vi "Convert Test Profile.vi"(0 "Test Profile":T5[](array[typedef]) {"Pump Cmds"."Pump 6\nCmd" min=0 format="%#.1f"; "Pump Cmds"."Pump 5\nCmd" min=0 format="%#.1f"; "Pump Cmds"."Pump 4\nCmd" min=0 format="%#.1f"; "Pump Cmds"."Pump 3\nCmd" min=0 format="%#.1f"; "Pump Cmds"."Pump 2\nCmd" min=0 format="%#.1f"; "Pump Cmds"."Pump 1\nCmd" min=0 format="%#.1f"; "Temp\nCmd" min=-60 max=100; "Pressure\nCmd" max=20; "PS\nCmd" min=0 max=20 format="%#.2f"; "Time (s)" min=0.0 step=0.01 format="%#.2g"}, 5 "App Config":T7={"Location"="", "Profiles Path"=path "", "Current Profile"="", "CA Number"="", "Controller Type:"=enum."Kuhnke", "Stagger Time (ms)"=0, "Tank 1 Fuel"="", "Tank 2 Fuel"="", "Serial Numbers"={"Position 1 SN"="", "Position 2 SN"="", "Poaition 3 SN"="", "Position 4 SN"="", "Position 5 SN"="", "Position 6 SN"=""}, "Pumps Present"={"Pump 1"=FALSE, "Pump 2"=FALSE, "Pump 3"=FALSE, "Pump 4"=FALSE, "Pump 5"=FALSE, "Pump 6"=FALSE}, "VoltCtrlRef"="", "VoltageSelect"=FALSE, "Watlow Present"=FALSE, "Temp 1"=0, "Temp 2"=0, "Voltage Scale"={"V_FFm"=10.0, "V_FFb"=0.0}, "Pressure Scale"={"Pres_FFm"=0.0, "Pres_FFb"=0.0}, "Temp Format"=0, "Temp Tolerance"=0.0, "Target Voltage"=0.0, "Target Pressure"=0.0, "Data Log Init"={"Data Path"=path "", "Data Log Rate (S/s)"=0, "AKLH Rate (Hours/S)"=0.0, "Sync Time Offset (min)"=0, "IP Last 3"=0, "WebDAV IP"=""}, "Email Handler IP"="", "ADC Check"=FALSE, "3 Pump Tank"=FALSE, "Freq Flow?"=FALSE, "Profile Temp Control"=FALSE, "Read Controller Diag"=FALSE, "FFT Min Freq."=0, "FFT Max Freq."=0, "Speed by Current"=FALSE, "Watlow is F4T?"=FALSE, "Test Stop Time"=0.0, "Stop Time Enable"=TRUE, "Timers Include Off-Time"=FALSE, "Pump Timer Email"={"Enable"=FALSE, "Hour to Send"=0}}, 7 "Controller Config":T1) -> (4 "Test Profile (FPGA)":T4[](array[typedef]))   [LabVIEW 2019]
uses:
  Type Defs/App Config.ctl
  Type Defs/Controller Names.ctl
  Data Logger/Data Log Init.ctl
  Type Defs/Pump Timer Email.ctl
  Type Defs/Test Step.ctl
  Type Defs/Pump Cmds.ctl
  Type Defs/Test Step (FPGA).ctl
  Controls/Controller Config.ctl
  Type Defs/Diagnostic Mode.ctl
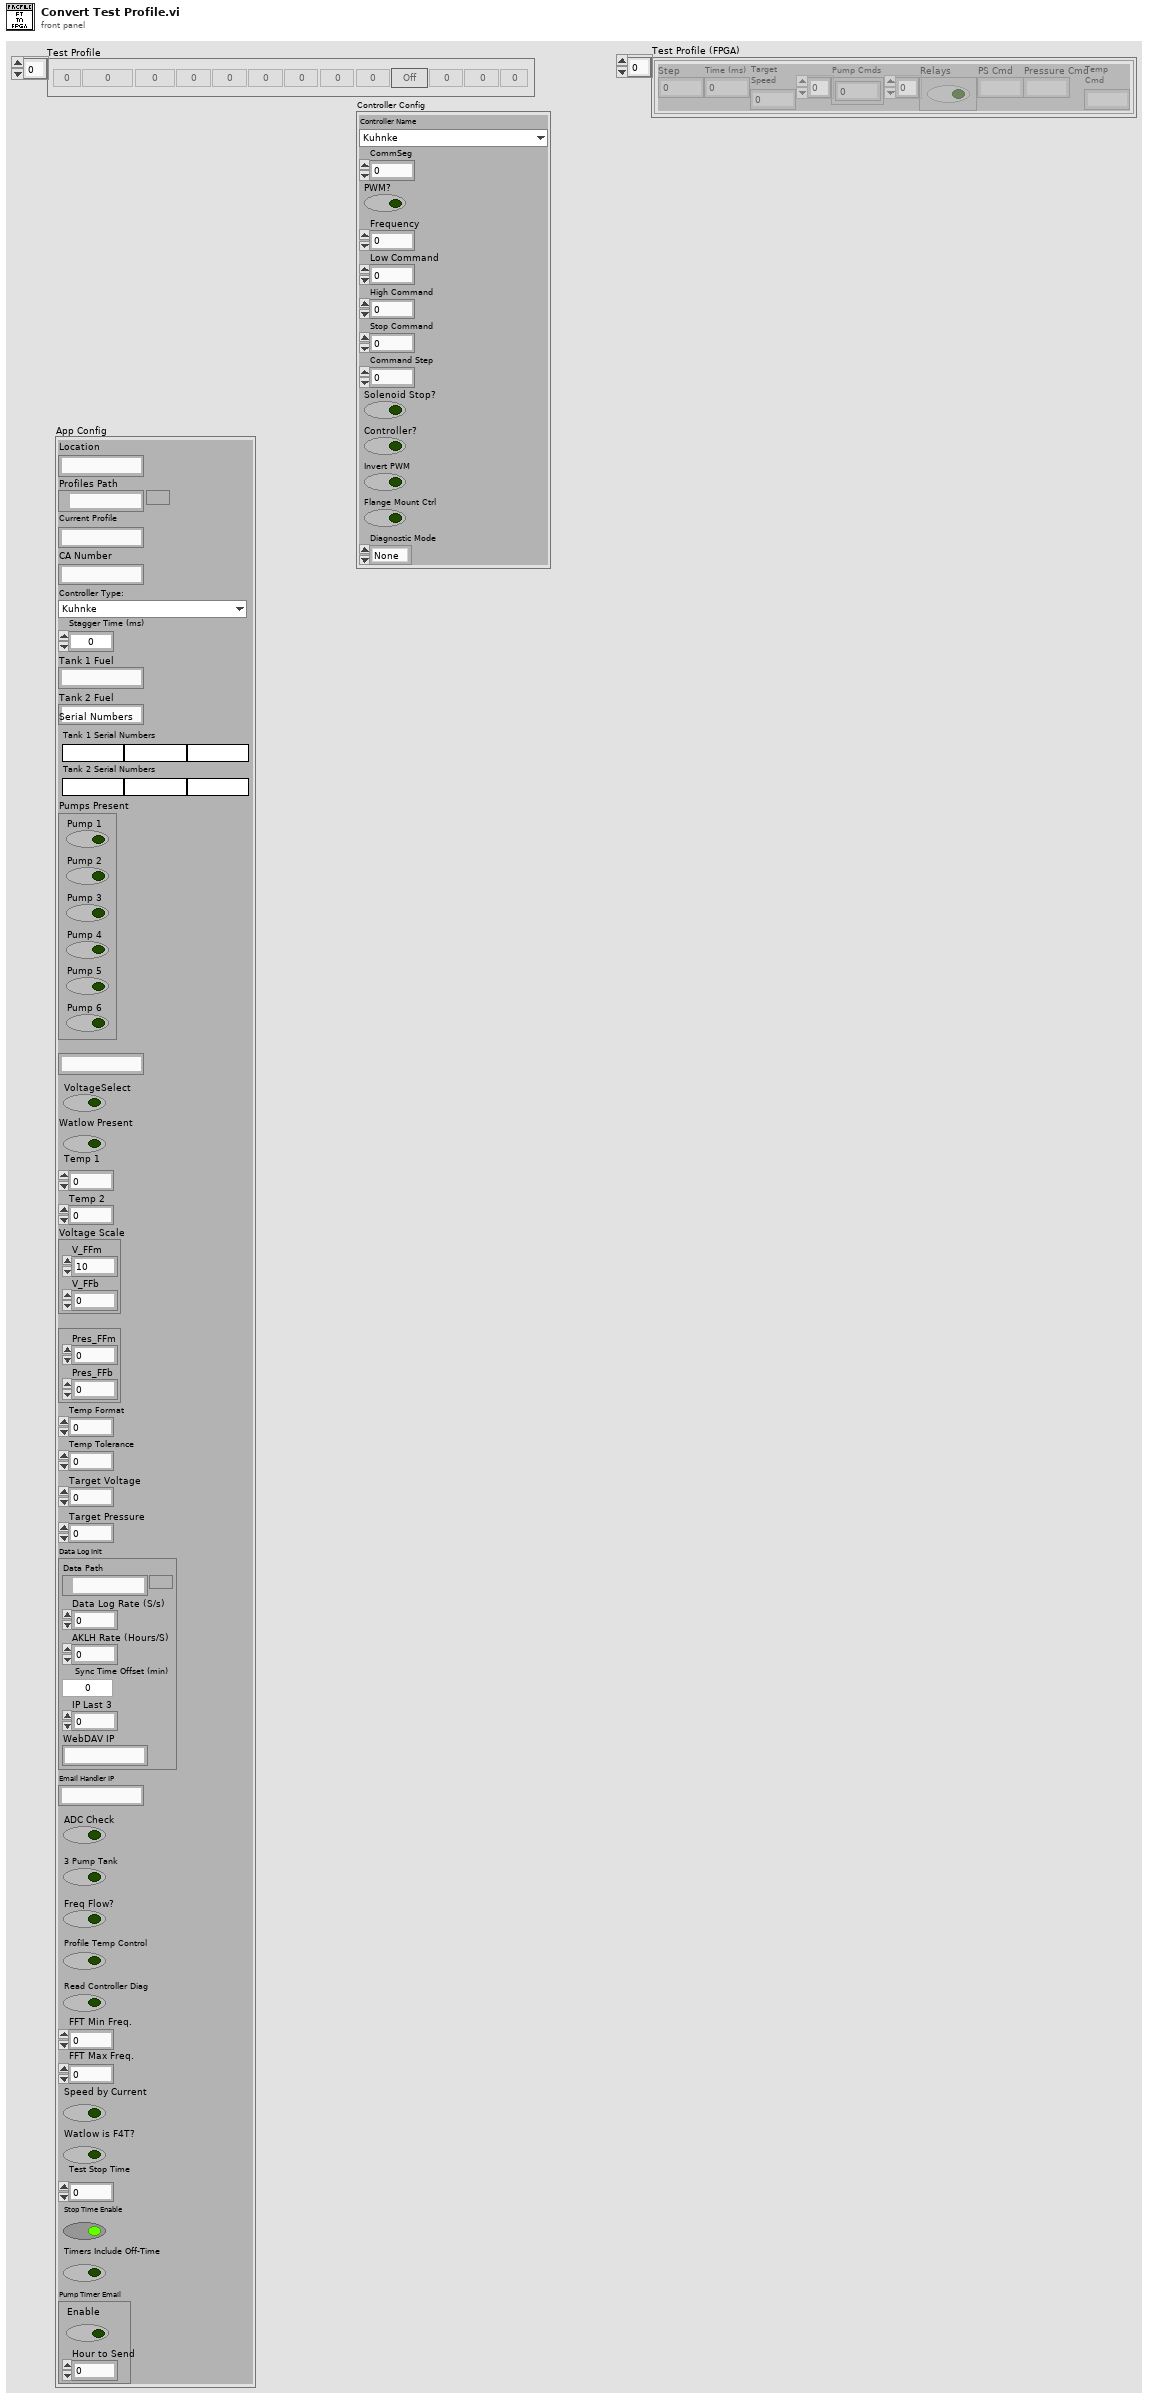
[diagram p1: front panel]
types:
  T1 = typedef "Controller Config.ctl" = cluster{"Controller Name":T2, "CommSeg":i32, "PWM?":bool, "Frequency":i32, "Low Command":dbl, "High Command":dbl, "Stop Command":dbl, "Command Step":dbl, "Solenoid Stop?":bool, "Controller?":bool, "Invert PWM":bool, "Flange Mount Ctrl":bool, "Diagnostic Mode":T3}
  T2 = typedef "Controller Names.ctl" = enum16{"Kuhnke", "Helbako BLDC", "Conti", "Hella BLDC OL PWM", "Hella BLDC Turbine OL PWM", "Hella BLDC Pressure", "Helbako (old)", "TI PWM", "PSA", "Hella Gas", "Hella Diesel", "8 Comm", "10 Comm", "8 Comm Hella", "10 Comm Hella", "8 Comm Omron", "10 Comm Omron", "8 Comm Nissan", "10 Comm Nissan", "8 Comm Hella (for FCA)", "Mazda BLDC", "CMFB"}
  T3 = typedef "Diagnostic Mode.ctl" = enum16{"None", "PSA", "CMFB"}
  T4 = typedef "Test Step (FPGA).ctl" = cluster{"Step":u8, "Time (ms)":u32, "Target\nSpeed":u16, "Pump Cmds":i32[], "Relays":bool[], "PS Cmd":fxp<+/-,20,5>, "Pressure Cmd":fxp<+/-,20,5>, "Temp\nCmd":i16}
  T5 = typedef "Test Step.ctl" = cluster{"Step":u8, "Time (s)":dbl, "Target\nSpeed":u16, "Pump Cmds":T6, "Relays":bool, "PS\nCmd":sgl, "Pressure\nCmd":u16, "Temp\nCmd":i16}
  T6 = typedef "Pump Cmds.ctl" = cluster{"Pump 1\nCmd":sgl, "Pump 2\nCmd":sgl, "Pump 3\nCmd":sgl, "Pump 4\nCmd":sgl, "Pump 5\nCmd":sgl, "Pump 6\nCmd":sgl}
  T7 = typedef "App Config.ctl" = cluster{"Location":string, "Profiles Path":path, "Current Profile":string, "CA Number":string, "Controller Type:":T2, "Stagger Time (ms)":i32, "Tank 1 Fuel":string, "Tank 2 Fuel":string, "Serial Numbers":cluster{"Position 1 SN":string, "Position 2 SN":string, "Poaition 3 SN":string, "Position 4 SN":string, "Position 5 SN":string, "Position 6 SN":string}, "Pumps Present":cluster{"Pump 1":bool, "Pump 2":bool, "Pump 3":bool, "Pump 4":bool, "Pump 5":bool, "Pump 6":bool}, "VoltCtrlRef":string, "VoltageSelect":bool, "Watlow Present":bool, "Temp 1":i16, "Temp 2":i16, "Voltage Scale":cluster{"V_FFm":dbl, "V_FFb":dbl}, "Pressure Scale":cluster{"Pres_FFm":dbl, "Pres_FFb":dbl}, "Temp Format":i32, "Temp Tolerance":dbl, "Target Voltage":dbl, "Target Pressure":dbl, "Data Log Init":T8, "Email Handler IP":string, "ADC Check":bool, "3 Pump Tank":bool, "Freq Flow?":bool, "Profile Temp Control":bool, "Read Controller Diag":bool, "FFT Min Freq.":i32, "FFT Max Freq.":i32, "Speed by Current":bool, "Watlow is F4T?":bool, "Test Stop Time":dbl, "Stop Time Enable":bool, "Timers Include Off-Time":bool, "Pump Timer Email":T9}
  T8 = typedef "Data Log Init.ctl" = cluster{"Data Path":path, "Data Log Rate (S/s)":u32, "AKLH Rate (Hours/S)":dbl, "Sync Time Offset (min)":i32, "IP Last 3":i32, "WebDAV IP":string}
  T9 = typedef "Pump Timer Email.ctl" = cluster{"Enable":bool, "Hour to Send":u8}
  T10 = cluster{"Pump 1":bool, "Pump 2":bool, "Pump 3":bool, "Pump 4":bool, "Pump 5":bool, "Pump 6":bool}
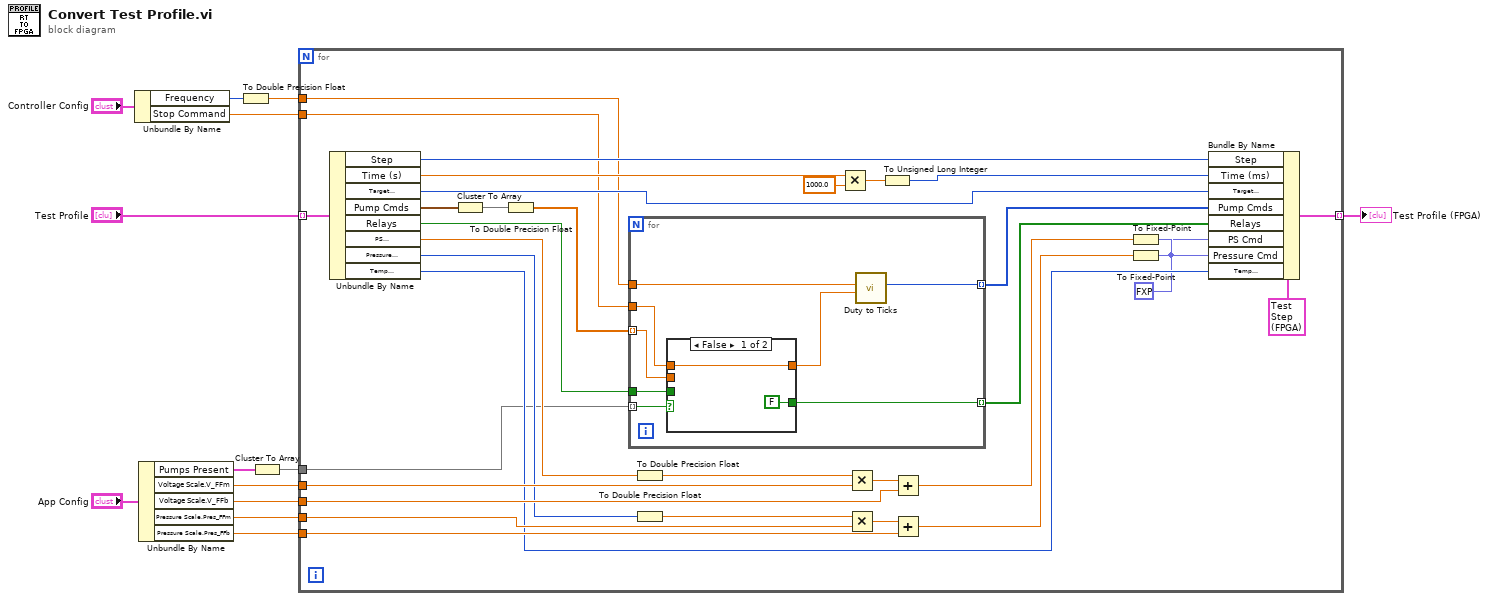
[diagram p0: block diagram]
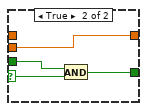
[diagram p2: hidden frame]
diagram:
  n1 = Unbundle By Name("Controller Config") -> ("Frequency"=w5:i32, "Stop Command"=w1:dbl)
  n2 = Unbundle By Name("App Config") -> ("Pumps Present"=w3:T10, "Voltage Scale.V_FFm"=w12:dbl, "Voltage Scale.V_FFb"=w11:dbl, "Pressure Scale.Pres_FFm"=w10:dbl, "Pressure Scale.Pres_FFb"=w9:dbl)
  n3 = To Double Precision Float(number=w5) -> (double precision float=w4:dbl)
  n4 = Cluster To Array(cluster=w3) -> (array=w2:bool[])
  n5 = for {
    tunnel: w12 -> [w39]
    tunnel: w11 -> [w36]
    tunnel: w10 -> [w32]
    tunnel: w9 -> [w31]
    tunnel: "Test Profile" -> [w27] mode=indexing
    tunnel: [w26] -> w7 mode=indexing
    tunnel: w4 -> [w18]
    tunnel: w2 -> [w16]
    tunnel: w1 -> [w15]
    w23 = fxp<+/-,20,5> 0.0 ("AO0")
    n6 = Unbundle By Name(w27) -> ("Step"=w47:u8, "Time (s)"=w46:dbl, "Target\nSpeed"=w30:u16, "Pump Cmds"=w42:T6, "Relays"=w17:bool, "PS\nCmd"=w40:sgl, "Pressure\nCmd"=w33:u16, "Temp\nCmd"=w29:i16)
    n7 = Cluster To Array(cluster=w42) -> (array=w20:sgl[])
    n8 = To Double Precision Float(number=w20) -> (double precision float=w41:dbl[])
    n9 = for {
      tunnel: w18 -> [w50]
      tunnel: w41 -> [w54] mode=indexing
      tunnel: [w48] -> w19 mode=indexing
      tunnel: w17 -> [w53]
      tunnel: w16 -> [w55] mode=indexing
      tunnel: w15 -> [w51]
      tunnel: [w52] -> w14 mode=indexing
      n10 = case shown="False" w55 {
        selector: w55 -> [_ w59]
        tunnel: w54 -> [_ w61]
        tunnel: [w56 w61] -> w49
        tunnel: w53 -> [_ w60]
        tunnel: [FALSE w58] -> w52
        tunnel: w51 -> [w56 _]
        frame False {
        }
        frame True {
          n11 = And(x=w60, y=w59) -> (x .and. y?=w58:bool)
        }
      }
      n12 = call "Duty to Ticks.vi"("Duty"=w49, "Frequency"=w50) -> ("Ticks"=w48:i32)  [unwired: 9 in]
    }
    n13 = To Double Precision Float(number=w40) -> (double precision float=w38:dbl)
    n14 = To Double Precision Float(number=w33) -> (double precision float=w34:dbl)
    n15 = Multiply(x=w46, y=1000.0) -> (x*y=w44:dbl)
    n16 = Multiply(x=w38, y=w39) -> (x*y=w37:dbl)
    n17 = Multiply(x=w34, y=w32) -> (x*y=w35:dbl)
    n18 = To Unsigned Long Integer(number=w44) -> (unsigned 32bit integer=w43:u32)
    n19 = Add(x=w37, y=w36) -> (x+y=w25:dbl)
    n20 = Add(x=w35, y=w31) -> (x+y=w24:dbl)
    n21 = To Fixed-Point(fixed-point type=w23, number=w25) -> (fixed-point=w22:fxp<+/-,20,5>)
    n22 = To Fixed-Point(fixed-point type=w23, number=w24) -> (fixed-point=w21:fxp<+/-,20,5>)
    n23 = Bundle By Name(cluster=T4 {"Step"=0, "Time (ms)"=0, "Target\nSpeed"=0, "Pump Cmds"=[0, 0, 0, 0, 0, 0], "Relays"=[FALSE, FALSE, FALSE, FALSE, FALSE, FALSE], "PS Cmd"=0.0, "Pressure Cmd"=0.0, "Temp\nCmd"=0} ("Test Step (FPGA)"), "Step"=w47, "Time (ms)"=w43, "Target\nSpeed"=w30, "Pump Cmds"=w19, "Relays"=w14, "PS Cmd"=w22, "Pressure Cmd"=w21, "Temp\nCmd"=w29) -> (w26:T4)
  }
  "Test Profile (FPGA)" <- w7
